vi "Begin.vi"(8 "error in":errorcluster) -> (0 "error out":errorcluster)   [LabVIEW 2023]
doc: "Called before other user functions, this VI can be used to open I/O refnums, load in file data, and do general program initialization. Notice that the <B>error out</B> terminal is simply used for data flow. Wiring it to other structures or subVIs ensures that this VI runs first."
uses:
  <vilib>/Rock Robotics/WPI/DriverStation/WPI_DriverStationRobotMode2.ctl
  <vilib>/Rock Robotics/WPI/Joystick/WPI_JoystickDeviceEnum.ctl
  Robot Global Data.vi
  <vilib>/Rock Robotics/Network Tables/NT Write String Array.vi
  <vilib>/Rock Robotics/WPI/SafetyOutput/WPI_SafetyOutputConfigMenu.ctl
  <vilib>/Rock Robotics/WPI/ThirdParty/REV Robotics/REVLib/Typedef/Spark MAX Idle Mode.ctl
  <vilib>/Rock Robotics/WPI/ThirdParty/REV Robotics/REVLib/Typedef/Spark MAX Sensor Type.ctl
panel:
  in  "Swerve Rotation PID":T1={"P Gain"=1.1, "I Gain"=0.0, "D Gain"=0.0, "F Gain"=0.0, "I Zone"=0.0, "Min Output"=-1.0, "Max Output"=1.0}
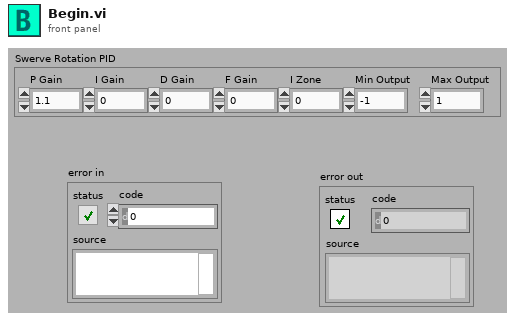
[diagram p1: front panel]
types:
  T1 = cluster{"P Gain":dbl, "I Gain":dbl, "D Gain":dbl, "F Gain":dbl, "I Zone":dbl, "Min Output":dbl, "Max Output":dbl}
  T2 = typedef "WPI_JoystickDeviceEnum.ctl" = enum16{"USB 0", "USB 1", "USB 2", "USB 3", "USB 4", "USB 5"}
  T3 = typedef "Spark MAX Sensor Type.ctl" = enum16{"No Sensor", "Hall Sensor", "Encoder", "-Not Available-", "Analog", "Alternate Encoder", "Duty Cycle"}
  T4 = typedef "Spark MAX Idle Mode.ctl" = enum16{"Coast", "Brake"}
  T5 = typedef "WPI_SafetyOutputConfigMenu.ctl" = enum16{"Enable", "Disable"}
  T6 = typedef "WPI_DriverStationRobotMode2.ctl" = enum16{"Autonomous Disabled", "Autonomous Enabled", "Teleop Disabled", "Teleop Enabled", "Disconnected", "Finish", "Test Disabled", "Test Enabled", "Emergency Stopped"}
  T7 = typedef "WPI_JoystickDevRef.ctl" = cluster{"Device":T2}
  T8 = typedef "ADIS16470 Device Reference.ctl" = cluster{"DevStatus":errorcluster, "Hardware Config":T9, "Calibration Complete":refnum<notifier>, "Status Reference":refnum<data-value>, "Data Reference":refnum<data-value>, "Sychronous Process VI":T13, "Cmd FIFO":refnum<k33>, "Source":T14, "Data FIFO":refnum<k33>, "Calibration Time (ms)":u32, "Data Reference":refnum<data-value>}
  T9 = typedef "ADIS16470 Hardware Configuration.ctl" = cluster{"SPI Clock Rate (Hz)":dbl, "IMU SPI Mode (3)":T10, "IMU Reset Pin":T11, "IMU SPI Bus":T12, "IMU Data Ready Pin":T11, "Stall Config":cluster{"Pow2BytesPerRead":u8, "StallTicks":u16, "CsToSclkTicks":u8}}
  T10 = typedef "WPI_SPIMode.ctl" = enum16{"Mode 0 (Clk Idle Low,Sample on Leading)", "Mode 1 (Clk Idle Low,Sample on Trailing)", "Mode 2 (Clk Idle High,Sample on Leading)", "Mode 3 (Clk Idle High,Sample on Trailing)"}
  T11 = typedef "FPGA_DIOChannel.ctl" = enum8{"DIO 0", "DIO 1", "DIO 2", "DIO 3", "DIO 4", "DIO 5", "DIO 6", "DIO 7", "DIO 8", "DIO 9", "DIO MXP 0", "DIO MXP 1", "DIO MXP 2", "DIO MXP 3", "DIO MXP 4", "DIO MXP 5", "DIO MXP 6", "DIO MXP 7", "DIO MXP 8", "DIO MXP 9", "DIO MXP 10", "DIO MXP 11", "DIO MXP 12", "DIO MXP 13", "DIO MXP 14", "DIO MXP 15", "SPI Port CS1", "SPI Port CS2", "SPI Port CS3", "SPI Port MISO", "SPI Port MOSI", "Invalid"}
  T12 = typedef "spi_bus.ctl" = enum16{"SPI On-Board, CS0", "SPI On-Board, CS1", "SPI On-Board, CS2", "SPI On-Board, CS3", "SPI MXP", "Invalid"}
  T13 = typedef "ADIS16470 Process.ctl" = refnum<vi>
  T14 = typedef "FPGA_CounterEncoderSourceConvertionLVSourceType.ctl" = cluster{"DevStatus":errorcluster, "AnalogTriggerMode?":bool, "DigitalMode":cluster{"DIO Channel":T15}, "AnalogTriggerMode":cluster{"AnalogTriggerIndex":T16, "OutputType":T17}}
  T15 = typedef "FPGA_DIODigitalSourceChannel.ctl" = enum8{"DIO 0", "DIO 1", "DIO 2", "DIO 3", "DIO 4", "DIO 5", "DIO 6", "DIO 7", "DIO 8", "DIO 9", "DIO MXP 0", "DIO MXP 1", "DIO MXP 2", "DIO MXP 3", "DIO MXP 4", "DIO MXP 5", "DIO MXP 6", "DIO MXP 7", "DIO MXP 8", "DIO MXP 9", "DIO MXP 10", "DIO MXP 11", "DIO MXP 12", "DIO MXP 13", "DIO MXP 14", "DIO MXP 15", "SPI Port CS1", "SPI Port CS2", "SPI Port CS3", "SPI Port MISO", "SPI Port MOSI", "Disabled"}
  T16 = typedef "FPGA_AnalogTriggerIndex.ctl" = enum8{"Trig 0", "Trig 1", "Trig 2", "Trig 3", "Trig 4", "Trig 5", "Trig 6", "Trig 7", "Invalid"}
  T17 = typedef "FPGA_AnalogTriggerOutType.ctl" = enum16{"InWindow", "TriggerState", "Rising", "Falling"}
  T18 = typedef "WPI_MotorControlDeviceRef.ctl" = cluster{"DeviceStatus":errorcluster, "Type":T19, "PWM":cluster{"PWM Channel":T20, "DeadBand":T21}, "CAN":cluster{"Device Number":u8, "SetOutput VI Ref":variant, "GetOutput VI Ref":variant, "Enable VI Ref":variant, "Disable VI Ref":variant, "Data":variant}, "Invert":bool, "DIO PWM":cluster{"PWM \"Enable\" Channel":T20, "DIOChannel":T11, "PWM Rate":dbl}}
  T19 = typedef "WPI_MotorControlType.ctl" = enum16{"PWM", "CAN", "DIO PWM"}
  T20 = typedef "FPGA_DIOPWMChannel.ctl" = enum8{"PWM 0", "PWM 1", "PWM 2", "PWM 3", "PWM 4", "PWM 5", "PWM 6", "PWM 7", "PWM 8", "PWM 9", "PWM MXP 0", "PWM MXP 1", "PWM MXP 2", "PWM MXP 3", "PWM MXP 4", "PWM MXP 5", "PWM MXP 6", "PWM MXP 7", "PWM MXP 8", "PWM MXP 9", "Invalid"}
  T21 = typedef "WPI_PWMDeadband.ctl" = cluster{"Name":string, "maxPositivePwm":i32, "minPositivePwm":i32, "centerPwm":i32, "maxNegativePwm":i32, "minNegativePwm":i32, "angularRange":u16}
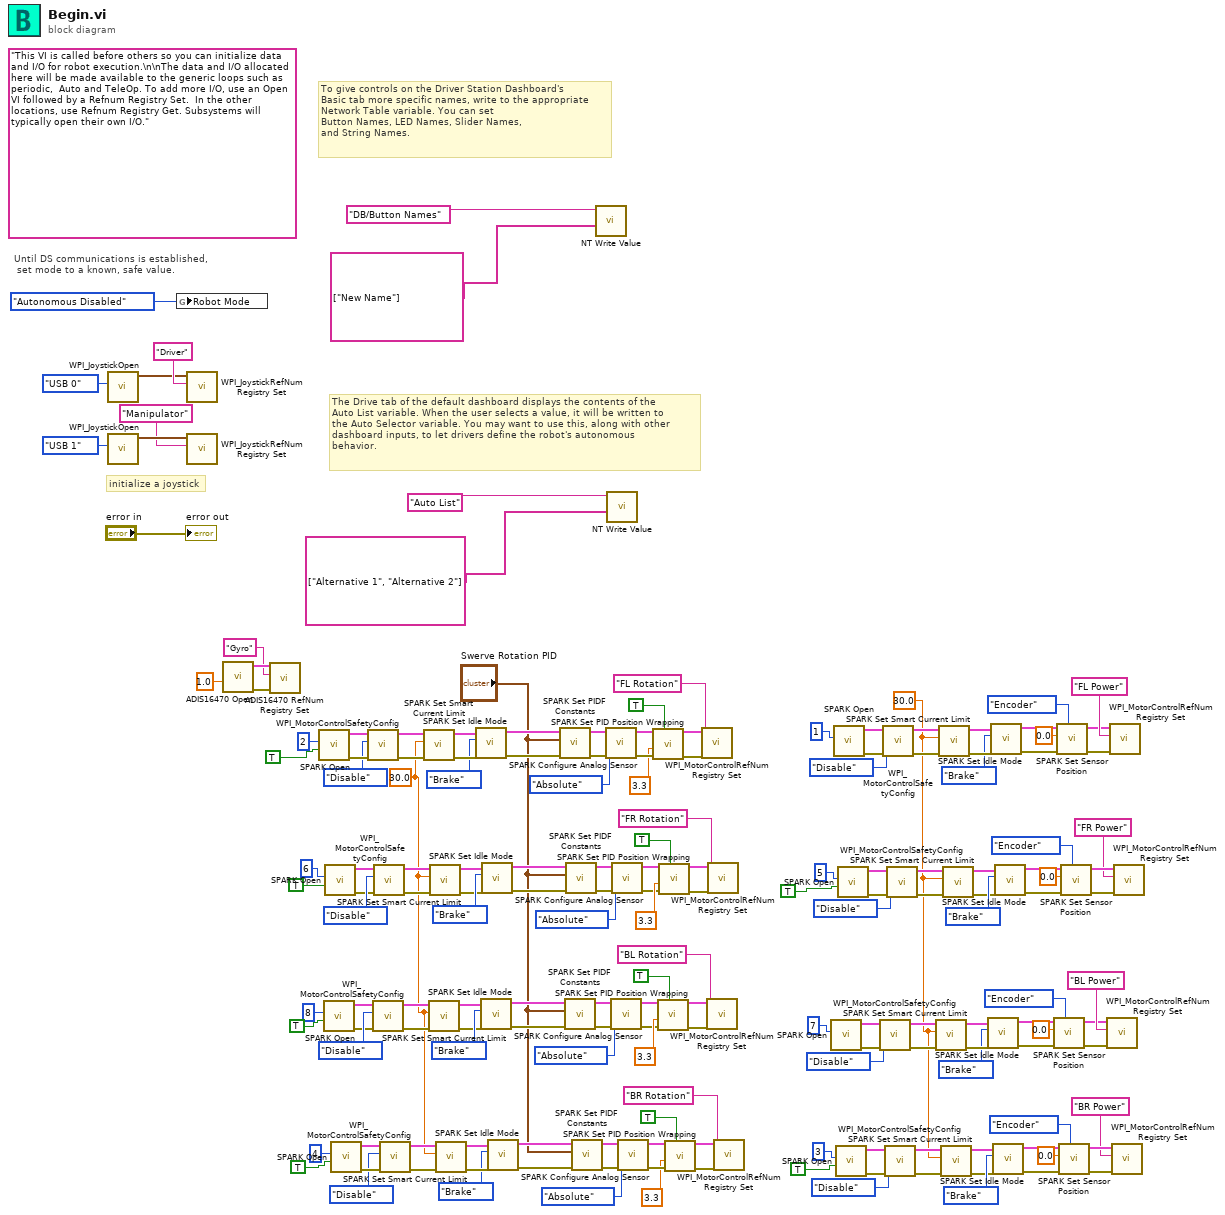
[diagram p0: block diagram]
diagram:
  w2 = 30.0 ("Primay Current Limit (80A)")
  w1 = 30.0 ("Primay Current Limit (80A)")
  (unwired) "This VI is called before others so you can initialize data and I/O for robot execution.\n\nThe data and I/O allocated here will be made available to the generic loops such as periodic,  Auto and TeleOp. To add more I/O, use an Open VI followed by a Refnum Registry Set.  In the other locations, use Refnum Registry Get. Subsystems will typically open their own I/O."
  # "The Drive tab of the default dashboard displays the contents of the\nAuto List variable. When the user selects a value, it will be written to\nthe Auto Selector variable. You may want to use this, along with other\ndashboard inputs, to let drivers define the robot's autonomous\nbehavior."
  # "To give controls on the Driver Station Dashboard's\nBasic tab more specific names, write to the appropriate\nNetwork Table variable. You can set\nButton Names, LED Names, Slider Names,\nand String Names."
  # "initialize a joystick"
  # "Until DS communications is established,\n set mode to a known, safe value."
  n1 = call <vilib>:"WPI_JoystickOpen.vi"("JoystickDevice"=WPI_JoystickDeviceEnum."USB 0") -> ("JoystickDevRef"=w171:T7)  [unwired: 10 in]
  n2 = call <vilib>:"WPI_JoystickOpen.vi"("JoystickDevice"=WPI_JoystickDeviceEnum."USB 1") -> ("JoystickDevRef"=w4:T7)  [unwired: 10 in]
  n3 = global write "Robot Global Data.vi" "Robot Mode"(WPI_DriverStationRobotMode2."Autonomous Disabled" ("Robot Mode")) -> ()
  n4 = call <vilib>:"WPI_JoystickRefNum Registry Set.vi"("refnum name"="Driver", "JoystickDevRef"=w171) -> ()  [unwired: 8 in, 2 out]
  n5 = call <vilib>:"WPI_JoystickRefNum Registry Set.vi"("refnum name"="Manipulator", "JoystickDevRef"=w4) -> ()  [unwired: 8 in, 2 out]
  n6 = call <vilib>:"ADIS16470 Open.vi"("Initial Calibration Time (4s)"=1.0) -> ("error out"=w9:errorcluster, "ADIS16470DevRef"=w8:T8)  [unwired: 9 in]
  n7 = call <vilib>:"ADIS16470 RefNum Registry Set.vi"("error in (no error)"=w9, "refnum name"="Gyro", "ADIS16470DevRef in"=w8) -> ()  [unwired: 7 in, 2 out]
  n8 = call <vilib>:"SPARK Open.vi"("Invert"=TRUE, "Device Number"=u8 2) -> ("error out"=w163:errorcluster, "MotorControlDeviceRef"=w162:T18)  [unwired: 8 in]
  n9 = call <vilib>:"SPARK Open.vi"("Invert"=TRUE, "Device Number"=u8 8) -> ("error out"=w82:errorcluster, "MotorControlDeviceRef"=w83:T18)  [unwired: 8 in]
  n10 = call <vilib>:"SPARK Open.vi"("Invert"=TRUE, "Device Number"=u8 6) -> ("error out"=w124:errorcluster, "MotorControlDeviceRef"=w125:T18)  [unwired: 8 in]
  n11 = call <vilib>:"SPARK Open.vi"("Invert"=TRUE, "Device Number"=u8 4) -> ("error out"=w121:errorcluster, "MotorControlDeviceRef"=w120:T18)  [unwired: 8 in]
  n12 = call <vilib>:"WPI_MotorControlSafetyConfig.vi"("error in (no error)"=w163, "mode"=WPI_SafetyOutputConfigMenu."Disable", "MotorControlDevRef"=w162) -> ("error out"=w160:errorcluster, "MotorControlDevRef"=w159:T18)  [unwired: 7 in]
  n13 = call <vilib>:"WPI_MotorControlSafetyConfig.vi"("error in (no error)"=w82, "mode"=WPI_SafetyOutputConfigMenu."Disable", "MotorControlDevRef"=w83) -> ("error out"=w85:errorcluster, "MotorControlDevRef"=w86:T18)  [unwired: 7 in]
  n14 = call <vilib>:"WPI_MotorControlSafetyConfig.vi"("error in (no error)"=w124, "mode"=WPI_SafetyOutputConfigMenu."Disable", "MotorControlDevRef"=w125) -> ("error out"=w127:errorcluster, "MotorControlDevRef"=w128:T18)  [unwired: 7 in]
  n15 = call <vilib>:"WPI_MotorControlSafetyConfig.vi"("error in (no error)"=w121, "mode"=WPI_SafetyOutputConfigMenu."Disable", "MotorControlDevRef"=w120) -> ("error out"=w118:errorcluster, "MotorControlDevRef"=w117:T18)  [unwired: 7 in]
  n16 = call <vilib>:"SPARK Set Smart Current Limit.vi"("error in (no error)"=w160, "Primay Current Limit (80A)"=w1, "MotorControlDeviceRef in"=w159) -> ("error out"=w158:errorcluster, "MotorControlDeviceRef out"=w157:T18)  [unwired: 7 in]
  n17 = call <vilib>:"SPARK Set Smart Current Limit.vi"("error in (no error)"=w85, "Primay Current Limit (80A)"=w1, "MotorControlDeviceRef in"=w86) -> ("error out"=w87:errorcluster, "MotorControlDeviceRef out"=w88:T18)  [unwired: 7 in]
  n18 = call <vilib>:"SPARK Set Smart Current Limit.vi"("error in (no error)"=w127, "Primay Current Limit (80A)"=w1, "MotorControlDeviceRef in"=w128) -> ("error out"=w129:errorcluster, "MotorControlDeviceRef out"=w130:T18)  [unwired: 7 in]
  n19 = call <vilib>:"SPARK Set Smart Current Limit.vi"("error in (no error)"=w118, "Primay Current Limit (80A)"=w1, "MotorControlDeviceRef in"=w117) -> ("error out"=w116:errorcluster, "MotorControlDeviceRef out"=w115:T18)  [unwired: 7 in]
  n20 = call <vilib>:"SPARK Set Idle Mode.vi"("error in (no error)"=w158, "Idle Mode"=Spark_MAX_Idle_Mode."Brake", "MotorControlDeviceRef in"=w157) -> ("error out"=w155:errorcluster, "MotorControlDeviceRef out"=w154:T18)  [unwired: 7 in]
  n21 = call <vilib>:"SPARK Set Idle Mode.vi"("error in (no error)"=w87, "Idle Mode"=Spark_MAX_Idle_Mode."Brake", "MotorControlDeviceRef in"=w88) -> ("error out"=w90:errorcluster, "MotorControlDeviceRef out"=w91:T18)  [unwired: 7 in]
  n22 = call <vilib>:"SPARK Set Idle Mode.vi"("error in (no error)"=w129, "Idle Mode"=Spark_MAX_Idle_Mode."Brake", "MotorControlDeviceRef in"=w130) -> ("error out"=w132:errorcluster, "MotorControlDeviceRef out"=w133:T18)  [unwired: 7 in]
  n23 = call <vilib>:"SPARK Set Idle Mode.vi"("error in (no error)"=w116, "Idle Mode"=Spark_MAX_Idle_Mode."Brake", "MotorControlDeviceRef in"=w115) -> ("error out"=w113:errorcluster, "MotorControlDeviceRef out"=w112:T18)  [unwired: 7 in]
  n24 = call <vilib>:"SPARK Set PIDF Constants.vi"("error in"=w155, "PID Constants"="Swerve Rotation PID", "MotorControlDeviceRef"=w154) -> ("error out"=w153:errorcluster, "MotorControlDeviceRef"=w152:T18)  [unwired: 7 in]
  n25 = call <vilib>:"SPARK Set PIDF Constants.vi"("error in"=w90, "PID Constants"="Swerve Rotation PID", "MotorControlDeviceRef"=w91) -> ("error out"=w92:errorcluster, "MotorControlDeviceRef"=w93:T18)  [unwired: 7 in]
  n26 = call <vilib>:"SPARK Set PIDF Constants.vi"("error in"=w132, "PID Constants"="Swerve Rotation PID", "MotorControlDeviceRef"=w133) -> ("error out"=w134:errorcluster, "MotorControlDeviceRef"=w135:T18)  [unwired: 7 in]
  n27 = call <vilib>:"SPARK Set PIDF Constants.vi"("error in"=w113, "PID Constants"="Swerve Rotation PID", "MotorControlDeviceRef"=w112) -> ("error out"=w111:errorcluster, "MotorControlDeviceRef"=w110:T18)  [unwired: 7 in]
  n28 = call-poly <vilib>:"NT Write Value.vi"("value"=string[] ["New Name"] ("String Array"), "name"="DB/Button Names" ("Name")) -> ()  [unwired: 9 in, 1 out]
  n29 = call <vilib>:"SPARK Configure Analog Sensor.vi"("error in (no error)"=w153, "Sensor Mode (Absolute)"=enum16{"Absolute", "Relative"}."Absolute", "MotorControlDeviceRef in"=w152) -> ("error out"=w150:errorcluster, "MotorControlDeviceRef"=w149:T18)  [unwired: 7 in]
  n30 = call-poly <vilib>:"NT Write Value.vi"("value"=string[] ["Alternative 1", "Alternative 2"] ("String Array"), "name"="Auto List" ("Name")) -> ()  [unwired: 9 in, 1 out]
  n31 = call <vilib>:"SPARK Configure Analog Sensor.vi"("error in (no error)"=w92, "Sensor Mode (Absolute)"=enum16{"Absolute", "Relative"}."Absolute", "MotorControlDeviceRef in"=w93) -> ("error out"=w95:errorcluster, "MotorControlDeviceRef"=w96:T18)  [unwired: 7 in]
  n32 = call <vilib>:"SPARK Configure Analog Sensor.vi"("error in (no error)"=w134, "Sensor Mode (Absolute)"=enum16{"Absolute", "Relative"}."Absolute", "MotorControlDeviceRef in"=w135) -> ("error out"=w137:errorcluster, "MotorControlDeviceRef"=w138:T18)  [unwired: 7 in]
  n33 = call <vilib>:"SPARK Configure Analog Sensor.vi"("error in (no error)"=w111, "Sensor Mode (Absolute)"=enum16{"Absolute", "Relative"}."Absolute", "MotorControlDeviceRef in"=w110) -> ("error out"=w108:errorcluster, "MotorControlDeviceRef"=w107:T18)  [unwired: 7 in]
  n34 = call <vilib>:"SPARK Set PID Position Wrapping.vi"("Enable (F)"=TRUE, "error in (no error)"=w150, "Maximum Output (0)"=3.3, "MotorControlDeviceRef in"=w149) -> ("error out"=w145:errorcluster, "MotorControlDeviceRef out"=w146:T18)  [unwired: 6 in]
  n35 = call <vilib>:"SPARK Set PID Position Wrapping.vi"("Enable (F)"=TRUE, "error in (no error)"=w95, "Maximum Output (0)"=3.3, "MotorControlDeviceRef in"=w96) -> ("error out"=w100:errorcluster, "MotorControlDeviceRef out"=w99:T18)  [unwired: 6 in]
  n36 = call <vilib>:"SPARK Set PID Position Wrapping.vi"("Enable (F)"=TRUE, "error in (no error)"=w137, "Maximum Output (0)"=3.3, "MotorControlDeviceRef in"=w138) -> ("error out"=w142:errorcluster, "MotorControlDeviceRef out"=w141:T18)  [unwired: 6 in]
  n37 = call <vilib>:"SPARK Set PID Position Wrapping.vi"("Enable (F)"=TRUE, "error in (no error)"=w108, "Maximum Output (0)"=3.3, "MotorControlDeviceRef in"=w107) -> ("error out"=w103:errorcluster, "MotorControlDeviceRef out"=w104:T18)  [unwired: 6 in]
  n38 = call <vilib>:"WPI_MotorControlRefNum Registry Set.vi"("error in (no error)"=w145, "refnum name"="FL Rotation", "MotorControlDevRef"=w146) -> ()  [unwired: 7 in, 2 out]
  n39 = call <vilib>:"WPI_MotorControlRefNum Registry Set.vi"("error in (no error)"=w100, "refnum name"="BL Rotation", "MotorControlDevRef"=w99) -> ()  [unwired: 7 in, 2 out]
  n40 = call <vilib>:"WPI_MotorControlRefNum Registry Set.vi"("error in (no error)"=w142, "refnum name"="FR Rotation", "MotorControlDevRef"=w141) -> ()  [unwired: 7 in, 2 out]
  n41 = call <vilib>:"WPI_MotorControlRefNum Registry Set.vi"("error in (no error)"=w103, "refnum name"="BR Rotation", "MotorControlDevRef"=w104) -> ()  [unwired: 7 in, 2 out]
  n42 = call <vilib>:"SPARK Open.vi"("Device Number"=u8 7) -> ("error out"=w42:errorcluster, "MotorControlDeviceRef"=w41:T18)  [unwired: 9 in]
  n43 = call <vilib>:"SPARK Open.vi"("Device Number"=u8 1) -> ("error out"=w78:errorcluster, "MotorControlDeviceRef"=w77:T18)  [unwired: 9 in]
  n44 = call <vilib>:"SPARK Open.vi"("Invert"=TRUE ("Enable (F)"), "Device Number"=u8 3) -> ("error out"=w13:errorcluster, "MotorControlDeviceRef"=w14:T18)  [unwired: 8 in]
  n45 = call <vilib>:"SPARK Open.vi"("Invert"=TRUE ("Enable (F)"), "Device Number"=u8 5) -> ("error out"=w45:errorcluster, "MotorControlDeviceRef"=w46:T18)  [unwired: 8 in]
  n46 = call <vilib>:"WPI_MotorControlSafetyConfig.vi"("error in (no error)"=w42, "mode"=WPI_SafetyOutputConfigMenu."Disable", "MotorControlDevRef"=w41) -> ("error out"=w39:errorcluster, "MotorControlDevRef"=w38:T18)  [unwired: 7 in]
  n47 = call <vilib>:"WPI_MotorControlSafetyConfig.vi"("error in (no error)"=w78, "mode"=WPI_SafetyOutputConfigMenu."Disable", "MotorControlDevRef"=w77) -> ("error out"=w75:errorcluster, "MotorControlDevRef"=w74:T18)  [unwired: 7 in]
  n48 = call <vilib>:"WPI_MotorControlSafetyConfig.vi"("error in (no error)"=w13, "mode"=WPI_SafetyOutputConfigMenu."Disable", "MotorControlDevRef"=w14) -> ("error out"=w16:errorcluster, "MotorControlDevRef"=w17:T18)  [unwired: 7 in]
  n49 = call <vilib>:"WPI_MotorControlSafetyConfig.vi"("error in (no error)"=w45, "mode"=WPI_SafetyOutputConfigMenu."Disable", "MotorControlDevRef"=w46) -> ("error out"=w48:errorcluster, "MotorControlDevRef"=w49:T18)  [unwired: 7 in]
  n50 = call <vilib>:"SPARK Set Smart Current Limit.vi"("error in (no error)"=w39, "Primay Current Limit (80A)"=w2, "MotorControlDeviceRef in"=w38) -> ("error out"=w37:errorcluster, "MotorControlDeviceRef out"=w36:T18)  [unwired: 7 in]
  n51 = call <vilib>:"SPARK Set Smart Current Limit.vi"("error in (no error)"=w75, "Primay Current Limit (80A)"=w2, "MotorControlDeviceRef in"=w74) -> ("error out"=w73:errorcluster, "MotorControlDeviceRef out"=w72:T18)  [unwired: 7 in]
  n52 = call <vilib>:"SPARK Set Smart Current Limit.vi"("error in (no error)"=w16, "Primay Current Limit (80A)"=w2, "MotorControlDeviceRef in"=w17) -> ("error out"=w18:errorcluster, "MotorControlDeviceRef out"=w19:T18)  [unwired: 7 in]
  n53 = call <vilib>:"SPARK Set Smart Current Limit.vi"("error in (no error)"=w48, "Primay Current Limit (80A)"=w2, "MotorControlDeviceRef in"=w49) -> ("error out"=w50:errorcluster, "MotorControlDeviceRef out"=w51:T18)  [unwired: 7 in]
  n54 = call <vilib>:"SPARK Set Idle Mode.vi"("error in (no error)"=w37, "Idle Mode"=Spark_MAX_Idle_Mode."Brake", "MotorControlDeviceRef in"=w36) -> ("error out"=w33:errorcluster, "MotorControlDeviceRef out"=w32:T18)  [unwired: 7 in]
  n55 = call <vilib>:"SPARK Set Idle Mode.vi"("error in (no error)"=w73, "Idle Mode"=Spark_MAX_Idle_Mode."Brake", "MotorControlDeviceRef in"=w72) -> ("error out"=w65:errorcluster, "MotorControlDeviceRef out"=w64:T18)  [unwired: 7 in]
  n56 = call <vilib>:"SPARK Set Idle Mode.vi"("error in (no error)"=w18, "Idle Mode"=Spark_MAX_Idle_Mode."Brake", "MotorControlDeviceRef in"=w19) -> ("error out"=w22:errorcluster, "MotorControlDeviceRef out"=w23:T18)  [unwired: 7 in]
  n57 = call <vilib>:"SPARK Set Idle Mode.vi"("error in (no error)"=w50, "Idle Mode"=Spark_MAX_Idle_Mode."Brake", "MotorControlDeviceRef in"=w51) -> ("error out"=w54:errorcluster, "MotorControlDeviceRef out"=w55:T18)  [unwired: 7 in]
  n58 = call <vilib>:"SPARK Set Sensor Position.vi"("Sensor Type (Hall Sensor)"=Spark_MAX_Sensor_Type."Encoder", "error in"=w33, "Position"=0.0, "MotorControlDeviceRef"=w32) -> ("error out"=w28:errorcluster, "MotorControlDeviceRef"=w29:T18)  [unwired: 6 in]
  n59 = call <vilib>:"SPARK Set Sensor Position.vi"("Sensor Type (Hall Sensor)"=Spark_MAX_Sensor_Type."Encoder", "error in"=w65, "Position"=0.0, "MotorControlDeviceRef"=w64) -> ("error out"=w60:errorcluster, "MotorControlDeviceRef"=w61:T18)  [unwired: 6 in]
  n60 = call <vilib>:"SPARK Set Sensor Position.vi"("Sensor Type (Hall Sensor)"=Spark_MAX_Sensor_Type."Encoder", "error in"=w22, "Position"=0.0, "MotorControlDeviceRef"=w23) -> ("error out"=w27:errorcluster, "MotorControlDeviceRef"=w26:T18)  [unwired: 6 in]
  n61 = call <vilib>:"SPARK Set Sensor Position.vi"("Sensor Type (Hall Sensor)"=Spark_MAX_Sensor_Type."Encoder", "error in"=w54, "Position"=0.0, "MotorControlDeviceRef"=w55) -> ("error out"=w59:errorcluster, "MotorControlDeviceRef"=w58:T18)  [unwired: 6 in]
  n62 = call <vilib>:"WPI_MotorControlRefNum Registry Set.vi"("error in (no error)"=w28, "refnum name"="BL Power", "MotorControlDevRef"=w29) -> ()  [unwired: 7 in, 2 out]
  n63 = call <vilib>:"WPI_MotorControlRefNum Registry Set.vi"("error in (no error)"=w60, "refnum name"="FL Power", "MotorControlDevRef"=w61) -> ()  [unwired: 7 in, 2 out]
  n64 = call <vilib>:"WPI_MotorControlRefNum Registry Set.vi"("error in (no error)"=w27, "refnum name"="BR Power", "MotorControlDevRef"=w26) -> ()  [unwired: 7 in, 2 out]
  n65 = call <vilib>:"WPI_MotorControlRefNum Registry Set.vi"("error in (no error)"=w59, "refnum name"="FR Power", "MotorControlDevRef"=w58) -> ()  [unwired: 7 in, 2 out]
  "error out" <- "error in"
